vi "CS POLARIS BME DG Client.ProcEvents.vi"(0 "i ref in":refnum<vi>, 5 "error in (no error)":errorcluster) -> (14 "i ref out":refnum<vi>, 19 "error out":errorcluster)   [LabVIEW 2009, in "CS POLARIS BME DG Client.lvlib"]
doc: "This method is used to define the events the object will listen to. Add your own events here."
uses:
  CS POLARIS BME DG Client.lvlib
  CSCore/BaseProcess/BaseProcess.event definition.ctl
  CSCore/CAEObj/CAEObj.event definition.ctl
  CSCore/BaseProcess/BaseProcess.descriptor string definition.ctl
  CSCore/BaseProcess/BaseProcess.lvlib
  CSCore/CAEObj/CAEObj.lvlib
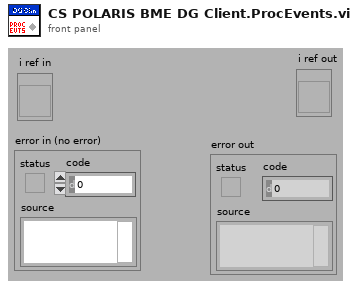
[diagram p1: front panel]
types:
  T1 = typedef "BaseProcess.lvlib/BaseProcess.event definition.ctl" = cluster{"CAEEvtDef":T2, "Data Descriptor":T3}
  T2 = typedef "CAEObj.lvlib/CAEObj.event definition.ctl" = cluster{"URL":string, "enable":bool, "ignoreResID":bool}
  T3 = typedef "BaseProcess.lvlib/BaseProcess.descriptor string definition.ctl" = string
  T4 = typedef "CS POLARIS BME DG Client.lvlib/CS POLARIS BME DG Client.i attribute.ctl" = cluster{"Delay Formula Ref":refnum<vi>, "Active Ref":refnum<vi>, "OutputModulo Ref":refnum<vi>, "Rep Rate Ref":refnum<vi>, "Next Shot Ref":refnum<vi>, "Error Ref":refnum<vi>, "Switch Ref":refnum<vi>, "New Delay Formula Ref":refnum<vi>, "New OutputModulo Ref ":refnum<vi>, "Channel":string, "CS DG Obj":string, "Stop Ref":refnum<vi>, "Max delay change":dbl, "Enabled fields":u8, "LockInfo Ref":refnum<vi>}
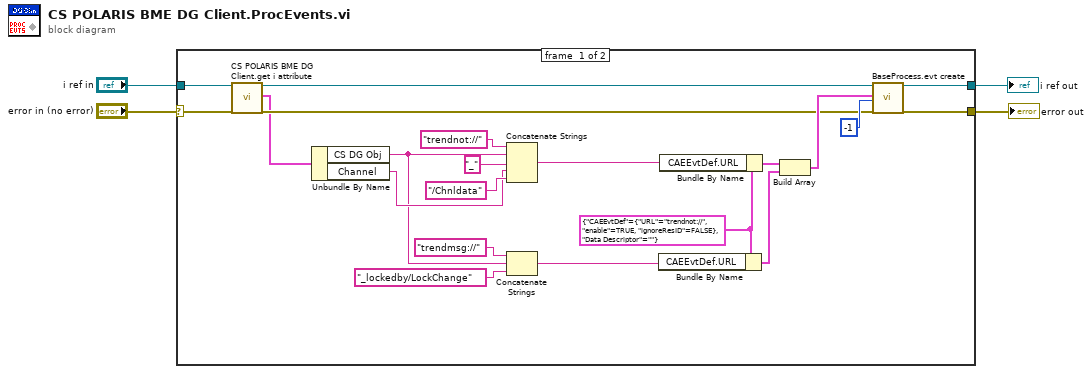
[diagram p0: block diagram]
diagram:
  n1 = case shown="No Error" "error in (no error)" {
    selector: "error in (no error)" -> [w17 w26]
    tunnel: "i ref in" -> [w15 w27]
    tunnel: [w25 w27] -> w3
    tunnel: [w24 w26] -> w2
    frame #0 {
      w10 = T1 {"CAEEvtDef"={"URL"="trendnot://", "enable"=TRUE, "ignoreResID"=FALSE}, "Data Descriptor"=""} ("Trigger")
      n2 = call "CS POLARIS BME DG Client.get i attribute.vi"("i ref in"=w15, "error in (no error)"=w17) -> ("i ref out"=w14:refnum<vi>, "i attribute"=w12:T4, "error out"=w16:errorcluster)  [unwired: 15 in]
      n3 = Unbundle By Name(w12) -> ("CS DG Obj"=w5:string, "Channel"=w9:string)
      n4 = Concatenate Strings("trendnot://" ("string"), w5, "_" ("string"), w9, "/Chnldata" ("string")) -> (w19:string)
      n5 = Concatenate Strings("trendmsg://" ("string"), w5, "_lockedby/LockChange" ("string")) -> (w7:string)
      n6 = Bundle By Name(cluster=w10, "CAEEvtDef.URL"=w7) -> (w6:T1)
      n7 = Bundle By Name(cluster=w10, "CAEEvtDef.URL"=w19) -> (w20:T1)
      n8 = Build Array(w20, w6) -> (w18:T1[])
      n9 = call "BaseProcess.evt create.vi"("i ref in"=w14, "newEvents"=w18, "ms timeout (10000)"=-1, "error in (no error)"=w16) -> ("i ref out"=w25:refnum<vi>, "error out"=w24:errorcluster)  [unwired: 12 in, 2 out]
    }
    frame #1 {
    }
  }
  "i ref out" <- w3
  "error out" <- w2
